vi "Dz from V.vi"(4 "data":variant, 5 "x":dbl) -> (2 "f(x)":dbl)   [LabVIEW 2015, in "DMA.lvclass"]
doc: "This VI serves as a template for solving for a diameter based on a given voltage."
uses:
  DMA.lvclass
  DMA.lvclass/DMA.ctl
  Particle Class/Particle Properties.lvclass/Particle Properties.ctl
  Particle Class/Accessors/Write D.vi
  Particle Class/Calculate Electric Mobility.vi
  Particle Class/Particle Properties.lvclass
panel:
  in  "error in":errorcluster
  out "error out":errorcluster
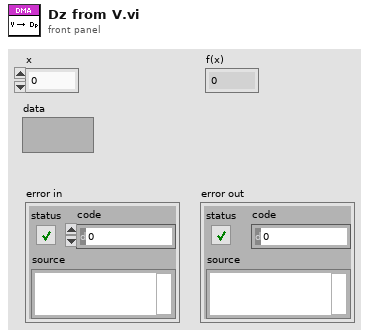
[diagram p1: front panel]
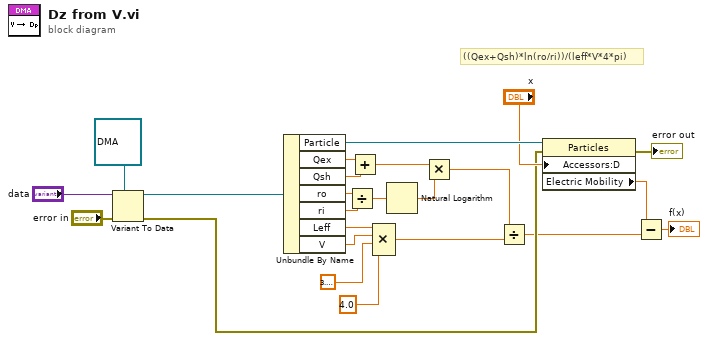
[diagram p0: block diagram]
diagram:
  # "((Qex+Qsh)*ln(ro/ri))/(leff*V*4*pi)"
  n1 = Variant To Data(error in="error in", type=refnum<class "DMA.lvclass"> refnum ("DMA"), Variant="data") -> (data=w11:refnum<class "DMA.lvclass">, error out=w8:errorcluster)
  n2 = Unbundle By Name(w11) -> ("Particle"=w22:refnum<class "Particle Properties.lvclass">, "Qex"=w16:dbl, "Qsh"=w15:dbl, "ro"=w14:dbl, "ri"=w13:dbl, "Leff"=w12:dbl, "V"=w10:dbl)
  n3 = Divide(x=w14, y=w13) -> (x/y=w21:dbl)
  n4 = Add(x=w16, y=w15) -> (x+y=w19:dbl)
  n5 = Compound Arithmetic op=MULTIPLY(w12, w10, 3.141592653589793, 4.0 ("x")) -> (w20:dbl)
  n6 = Natural Logarithm(1:w21) -> (0:w18:dbl)
  n7 = Multiply(x=w19, y=w18) -> (x*y=w17:dbl)
  n8 = Divide(x=w17, y=w20) -> (x/y=w5:dbl)
  n9 = property class="Particles"(reference=w22, error in=w8, "Accessors:D"="x") -> (error out=→"error out":errorcluster, "Electric Mobility"=w6:dbl)  [unwired: 1 out]
  n10 = Subtract(x=w6, y=w5) -> (x-y=→"f(x)":dbl)
